vi "User event test.vi"() -> ()   [LabVIEW 2021]
panel:
  in  "My user event":dbl
  out "number (0 to 1) 2":dbl
  out "number (0 to 1)":dbl
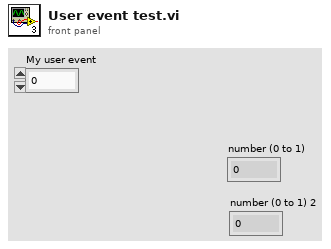
[diagram p1: front panel]
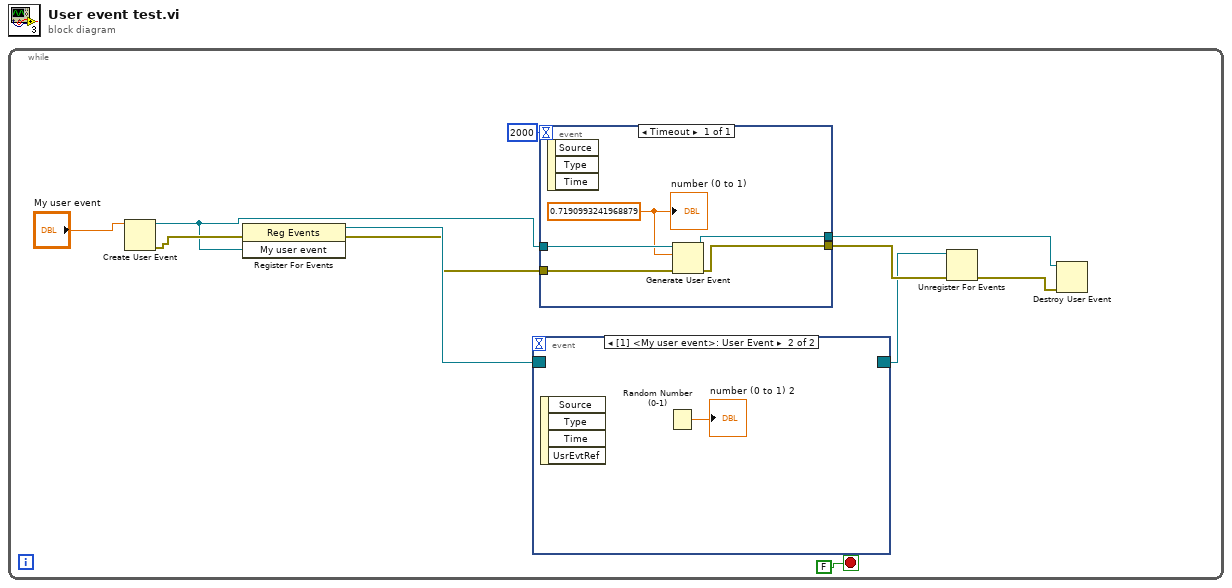
[diagram p0: block diagram]
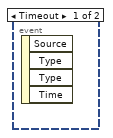
[diagram p2: hidden frame]
diagram:
  n1 = while {
    stop <- FALSE stop-if-true
    n2 = Create User Event(user event datatype="My user event") -> (user event=w4:refnum<user-event>, error out=w7:errorcluster)  [unwired: 1 in]
    n3 = register-events(error in=w7, w4) -> (reference out=w6:refnum<event-registration>, error out=w5:errorcluster)  [unwired: 1 in]
    n4 = event shown="[1] <My user event>: User Event" {
      selector: w6 -> [_ _]
      dyn-events: [_ _] -> w2
      timeout: _ -> [_ _]
      event Timeout {
        n5 = event-data() -> ()  [unwired: 1 in, 4 out]
      }
      event User Event {
        n6 = event-data() -> ()  [unwired: 1 in, 4 out]
        n7 = Random Number (0-1)() -> (number: 0 to 1=→"number (0 to 1) 2":dbl)
      }
    }
    n8 = event shown="[0] Timeout" {
      selector: _ -> [_]
      dyn-events: _ -> [_]
      timeout: 2000 -> [_]
      tunnel: w4 -> [w17]
      tunnel: w5 -> [w15]
      tunnel: [w14] -> w9
      tunnel: [w13] -> w1
      event Timeout {
        w16 = 0.7190993241968879 ("number (0 to 1)")
        n9 = event-data() -> ()  [unwired: 1 in, 3 out]
        n10 = Generate User Event(user event=w17, event data cluster=w16, error in=w15) -> (user event out=w13:refnum<user-event>, error out=w14:errorcluster)  [unwired: 1 in]
        "number (0 to 1)" <- w16
      }
    }
    n11 = Unregister For Events(event registration refnum=w2, error in=w9) -> (error out=w3:errorcluster)
    n12 = Destroy User Event(user event=w1, error in=w3) -> ()  [unwired: 1 out]
  }
